vi "zadanie 5.vi"() -> ()   [LabVIEW 2020]
uses:
  <vilib>/Analysis/3filter.llb/Filter Passband Type.ctl
  <vilib>/Analysis/4window.llb/windowTd.ctl
  <vilib>/Analysis/4window.llb/Gaussian Window (DBL).vi
  <vilib>/Analysis/3filter.llb/Butterworth Filter (DBL).vi
  <vilib>/Analysis/NI_AALBase.lvlib
  <vilib>/Analysis/NI_AALPro.lvlib
  <vilib>/gmath/NI_Gmath.lvlib
panel:
  in  "?":bool
  in  "?":bool
  in  "?":T1(tab)
  in  "Добавка":string(combo)
  out "График сигнала":dbl[](graph)
  in  "Вид сигнала":string(combo)
  in  "Вкл фильтр":bool
  in  "Тип фильтра":T2
  in  "Частота дискритизации: fs":dbl=1.0 format="%0.2f"
  in  "Верхняя частота среза: fh":dbl=0.45000000000000007 format="%0.2f"
  in  "Нижняя частота среза: fl":dbl=0.12500000000000006 format="%0.4f"
  in  "Порядок \nфильтра":i32=2
  out "Сигнал по фильтра":dbl[](graph)
  out "Спектр":T3(graph)
  in  "standard deviation":dbl=0.2
  out "Спектр с окном":T3(graph)
  in  "window info":cluster{"type":T4, "length":i32}={"type"=1, "length"=64} {"type" items=["Rectangle"=0, "Hanning"=1, "Hamming"=2, "Blackman-Harris"=3, "Exact Blackman"=4, "Blackman"=5, "Flat Top"=6, "4 Term B-Harris "=7, "7 Term B-Harris"=8, "Low Sidelobe"=9, "Blackman Nuttall"=11, "Triangle"=30, "Bartlett-Hanning"=31, "Bohman"=32, "Parzen"=33, "Welch"=34, "Kaiser"=60, "Dolph-Chebyshev"=61, "Gaussian"=62]}
  in  "time-freq sampling info":cluster{"time steps":i32, "frequency bins":i32}={"time steps"=-1, "frequency bins"=512}
  out "Спектограмма":dbl[][](graph)
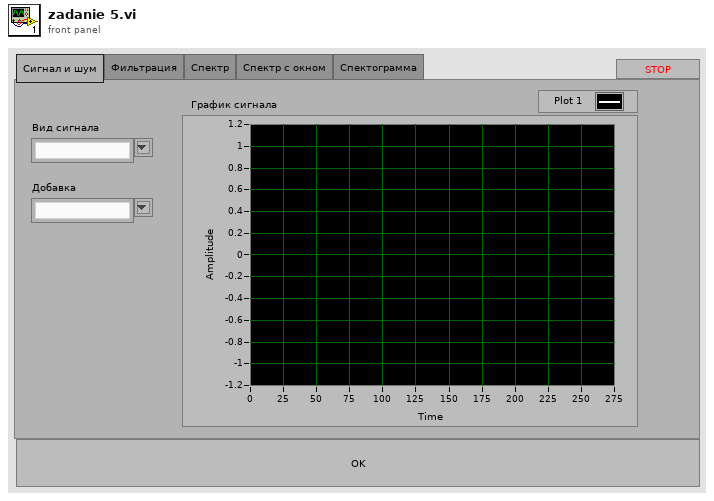
[diagram p1: front panel]
types:
  T1 = enum32{"Сигнал и шум", "Фильтрация", "Спектр", "Спектр с окном", "Спектограмма"}
  T2 = typedef "NI_AALBase.lvlib/Filter Passband Type.ctl" = enum32{"Lowpass", "Highpass", "Bandpass", "Bandstop"}
  T3 = cluster{dbl, "df":dbl, "Power Spectrum (V^2 rms)":dbl[]}
  T4 = typedef "NI_AALPro.lvlib/windowTd.ctl" = u32
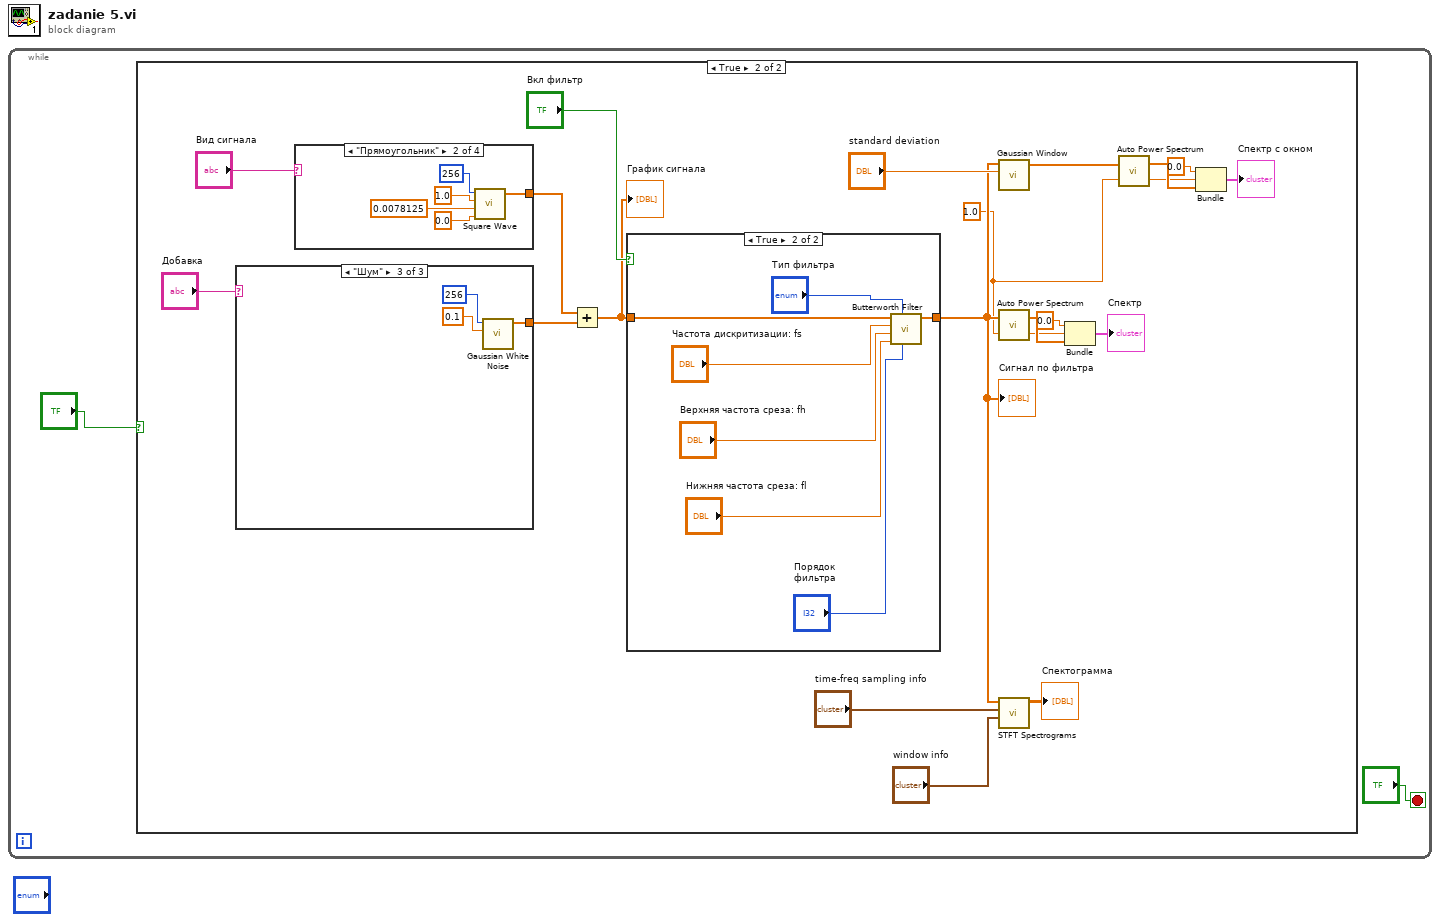
[diagram p0: block diagram]
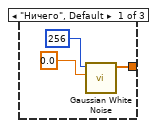
[diagram p4: hidden frame]
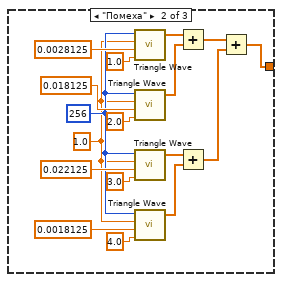
[diagram p5: hidden frame]
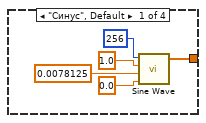
[diagram p6: hidden frame]
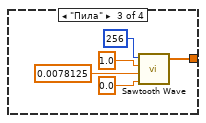
[diagram p7: hidden frame]
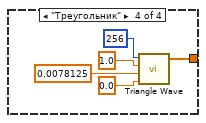
[diagram p8: hidden frame]
diagram:
  n1 = while {
    stop <- "?" stop-if-true
    n2 = case shown="True" "?" {
      frame False {
      }
      frame True {
        w5 = 1.0 ("dt")
        n3 = case shown="\"Шум\"" "Добавка" {
          tunnel: [w32 w35 w52] -> w22
          frame "Ничего", Default {
            n4 = call <vilib>:"Gaussian White Noise.vi"("standard deviation"=0.0, "samples"=256) -> ("Gaussian noise pattern"=w32:dbl[])  [unwired: 8 in, 1 out]
          }
          frame "Помеха" {
            w47 = 1.0 ("amplitude")
            w48 = 256 ("samples")
            n5 = call <vilib>:"Triangle Wave.vi"("samples"=w48, "amplitude"=w47, "frequency"=0.0028125, "phase in"=1.0) -> ("triangle wave"=w41:dbl[])  [unwired: 1 in, 2 out]
            n6 = call <vilib>:"Triangle Wave.vi"("samples"=w48, "amplitude"=w47, "frequency"=0.018125, "phase in"=2.0) -> ("triangle wave"=w40:dbl[])  [unwired: 1 in, 2 out]
            n7 = call <vilib>:"Triangle Wave.vi"("samples"=w48, "amplitude"=w47, "frequency"=0.022125, "phase in"=3.0) -> ("triangle wave"=w39:dbl[])  [unwired: 1 in, 2 out]
            n8 = call <vilib>:"Triangle Wave.vi"("samples"=w48, "amplitude"=w47, "frequency"=0.0018125, "phase in"=4.0) -> ("triangle wave"=w38:dbl[])  [unwired: 1 in, 2 out]
            n9 = Add(x=w41, y=w40) -> (x+y=w37:dbl[])
            n10 = Add(x=w39, y=w38) -> (x+y=w36:dbl[])
            n11 = Add(x=w37, y=w36) -> (x+y=w35:dbl[])
          }
          frame "Шум" {
            n12 = call <vilib>:"Gaussian White Noise.vi"("standard deviation"=0.1, "samples"=256) -> ("Gaussian noise pattern"=w52:dbl[])  [unwired: 8 in, 1 out]
          }
        }
        n13 = case shown="\"Прямоугольник\"" "Вид сигнала" {
          tunnel: [w55 w64 w69 w70] -> w23
          frame "Синус", Default {
            n14 = call <vilib>:"Sine Wave.vi"("samples"=256, "amplitude"=1.0, "frequency"=0.0078125, "phase in"=0.0) -> ("sine wave"=w55:dbl[])  [unwired: 1 in, 2 out]
          }
          frame "Прямоугольник" {
            n15 = call <vilib>:"Square Wave.vi"("samples"=256, "amplitude"=1.0, "frequency"=0.0078125, "phase in"=0.0) -> ("square wave"=w64:dbl[])  [unwired: 2 in, 2 out]
          }
          frame "Пила" {
            n16 = call <vilib>:"Sawtooth Wave.vi"("samples"=256, "amplitude"=1.0, "frequency"=0.0078125, "phase in"=0.0) -> ("sawtooth wave"=w69:dbl[])  [unwired: 1 in, 2 out]
          }
          frame "Треугольник" {
            n17 = call <vilib>:"Triangle Wave.vi"("samples"=256, "amplitude"=1.0, "frequency"=0.0078125, "phase in"=0.0) -> ("triangle wave"=w70:dbl[])  [unwired: 1 in, 2 out]
          }
        }
        n18 = Add(x=w23, y=w22) -> (x+y=w19:dbl[])
        "График сигнала" <- w19
        n19 = case shown="True" "Вкл фильтр" {
          tunnel: w19 -> [w24 w31]
          tunnel: [w24 w25] -> w12
          frame False {
          }
          frame True {
            n20 = call-poly <vilib>:"Butterworth Filter.vi"("order"="Порядок \nфильтра", "filter type"="Тип фильтра", "low cutoff freq: fl"="Нижняя частота среза: fl", "high cutoff freq: fh"="Верхняя частота среза: fh", "sampling freq: fs"="Частота дискритизации: fs", "X"=w31) -> ("Filtered X"=w25:dbl[])  [unwired: 2 in, 1 out]
          }
        }
        "Сигнал по фильтра" <- w12
        n21 = call-poly <vilib>:"Gaussian Window.vi"("standard deviation"="standard deviation", "X"=w12) -> ("Windowed X"=w4:dbl[])  [unwired: 8 in, 1 out]
        n22 = call <vilib>:"Auto Power Spectrum.vi"("dt"=w5, "Signal (V)"=w12) -> ("df"=w15:dbl, "Power Spectrum (V^2 rms)"=w16:dbl[])
        n23 = call <vilib>:"STFT Spectrograms.vi"("window info"="window info", "time-freq sampling info"="time-freq sampling info", "X"=w12) -> ("STFT Spectrogram {X}"=→"Спектограмма":dbl[][])  [unwired: 7 in, 1 out]
        n24 = Bundle(0.0, "df"=w15, "Power Spectrum (V^2 rms)"=w16) -> (→"Спектр":T3)  [unwired: 1 in]
        n25 = call <vilib>:"Auto Power Spectrum.vi"("dt"=w5, "Signal (V)"=w4) -> ("df"=w3:dbl, "Power Spectrum (V^2 rms)"=w11:dbl[])
        n26 = Bundle(0.0, "df"=w3, "Power Spectrum (V^2 rms)"=w11) -> (→"Спектр с окном":T3)  [unwired: 1 in]
      }
    }
  }
